vi "Mod_OFDM_Retrieve_Frame_Parameters.vi"(0 "Configuration in":variant, 11 "error in (no error)":errorcluster) -> (2 "Pulse Shaping Parameters":T2={"System Filter"={"TX Filter"=enum."Root Raised Cos", "Alpha"=0.5, "filter length"=8}, "Modulation system parameters"={"samples per symbol (16)"=16}, "symbol rate (Hz)"=1.0} {"symbol rate (Hz)" min=1.0 step=1.0 format="%.2p"; "Modulation system parameters"."samples per symbol (16)" step=2; "System Filter"."Alpha" min=0.0 max=1.0 step=0.05 format="%.2f"}, 4 "Parameters per Ofdm Symbol":T1 {"Data Source"."Data Source"."Register Initial State" format="%08x"}, 8 "Initial SEED IN":u32[](array[numeric]), 15 "error out":errorcluster)   [LabVIEW 2010]
doc: "The VI recovers the configuration settings from the variant into an array of clusters. The size of the array is the number of OFDM Symbols in the frame. Each cluster contains the configuration settings perataining to an OFDM symbol."
uses:
  Controls(Type_DEf)/Configure Pulse Shaping.ctl
  Controls(Type_DEf)/Parameters per Ofdm Symbol.ctl
  Polymorphic_Sub_VI's/Mod_OFDM_Get_OFDM_Frame.vi
  Polymorphic_Sub_VI's/Mod_OFDM_Get_Pulse_Shaping.vi
  Polymorphic_Sub_VI's/Mod_OFDM_Get_Data_Sources.vi
  Polymorphic_Sub_VI's/Mod_OFDM_Get_Modulator_Sources.vi
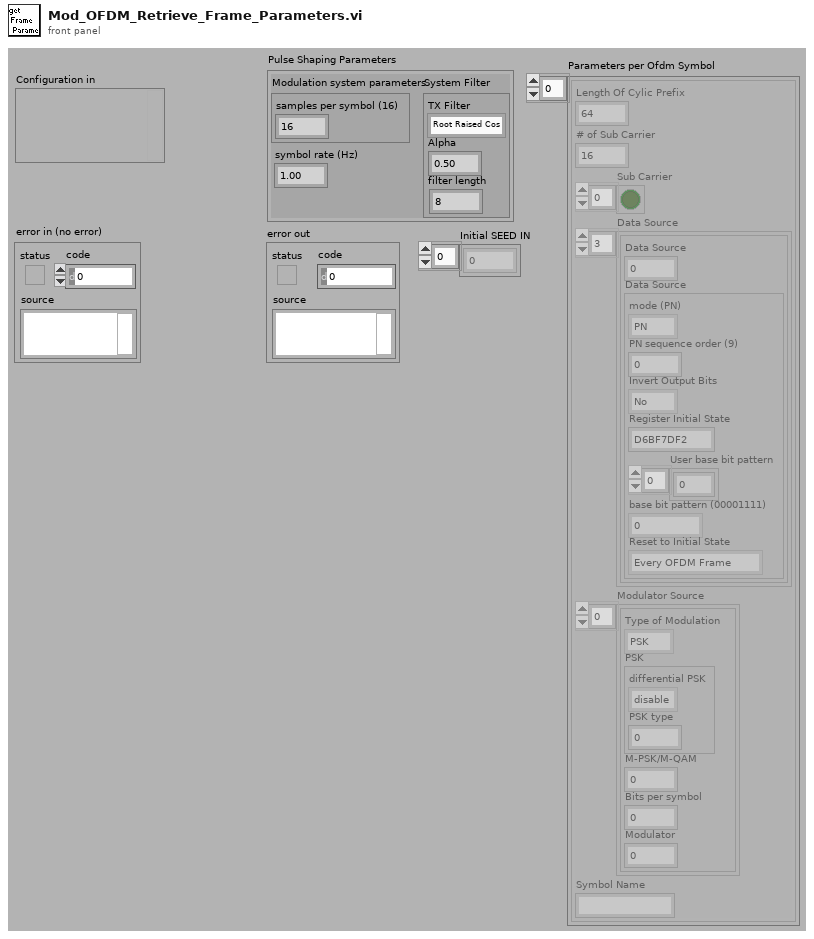
[diagram p1: front panel]
types:
  T1 = typedef "Parameters per Ofdm Symbol.ctl" = cluster{"Length Of Cylic Prefix":i32, "# of Sub Carrier":i32, "Sub Carrier":bool[], "Data Source":cluster{"Data Source":u16, "Data Source":cluster{"mode (PN)":enum16{"PN", "pattern", "user"}, "PN sequence order (9)":i32, "Invert Output Bits":enum16{"No", "Yes"}, "Register Initial State":u32, "User base bit pattern":i8[], "base bit pattern (00001111)":enum16{"0", "1", "01", "0011", "00001111"}, "Reset to Initial State":enum16{"Every OFDM Frame", "Every OFDM Symbol", "Every Sub Carrier"}}}[], "Modulator Source":cluster{"Type of Modulation":enum16{"PSK", "QAM"}, "PSK":cluster{"differential PSK":enum16{"disable", "enable"}, "PSK type":u16}, "M-PSK/M-QAM":i32, "Bits per symbol":i32, "Modulator":u16}[], "Symbol Name":string}[]
  T2 = typedef "Configure Pulse Shaping.ctl" = cluster{"System Filter":cluster{"TX Filter":enum16{"none", "Raised Cosine", "Root Raised Cos"}, "Alpha":dbl, "filter length":i32}, "Modulation system parameters":cluster{"samples per symbol (16)":u32}, "symbol rate (Hz)":dbl}
  T3 = cluster{"Symbol Name":string, "# of Symbols":i32}[]
  T4 = typedef "Pool of Data Source Control.ctl" = cluster{"mode (PN)":enum16{"PN", "pattern", "user"}, "PN sequence order (9)":i32, "Invert Output Bits":enum16{"No", "Yes"}, "Register Initial State ":u32, "User base bit pattern":i8[], "base bit pattern (00001111)":enum16{"0", "1", "01", "0011", "00001111"}, "Reset to Initial State":enum16{"Every OFDM Frame", "Every OFDM Symbol", "Every Sub Carrier"}}[]
  T5 = typedef "Pool of Modulator Control.ctl" = cluster{"M-QAM":enum16{"4", "16", "64", "256"}, "M-PSK":enum16{"2", "4", "8", "16", "32", "64", "128", "256"}, "Type of Modulation":enum16{"PSK", "QAM"}, " PSK":cluster{"differential PSK":enum16{"disable", "enable"}, "PSK type":enum16{"normal", "shifted", "offset"}}}[]
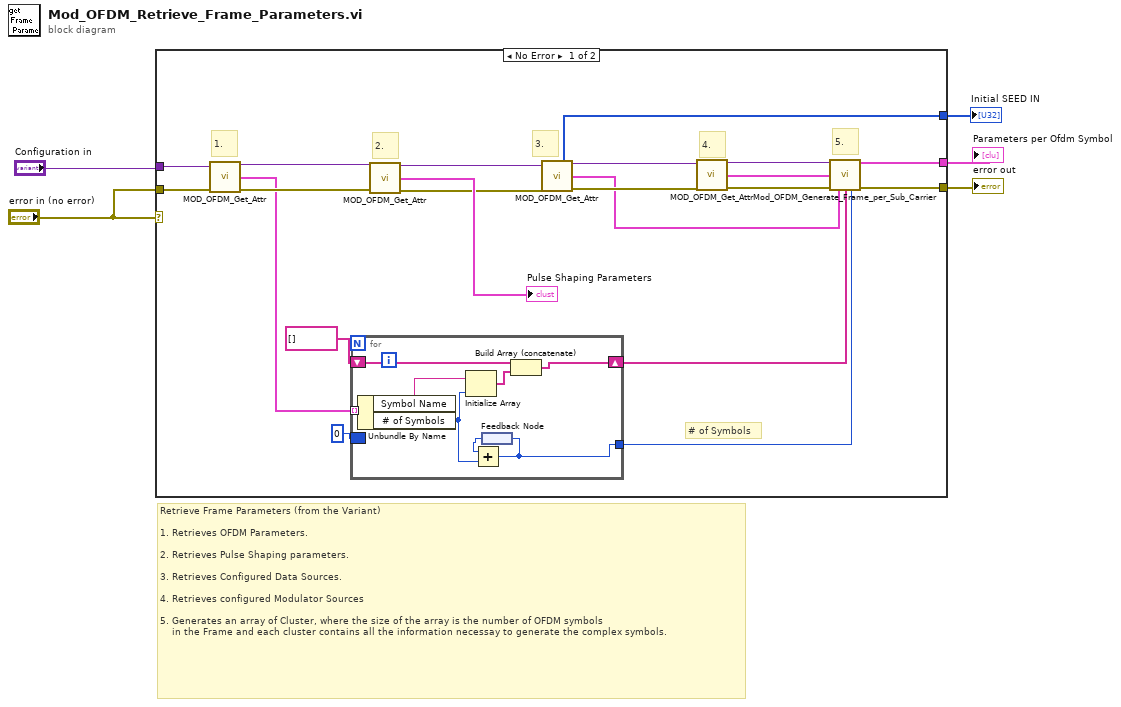
[diagram p0: block diagram]
diagram:
  # "Retrieve Frame Parameters (from the Variant)\n\n1. Retrieves OFDM Parameters.\n \n2. Retrieves Pulse Shaping parameters.\n\n3. Retrieves Configured Data Sources.\n\n4. Retrieves configured Modulator Sources\n\n5. Generates an array of Cluster, where the size of the array is the number of OFDM symbols\n    in the Frame and each cluster contains all the information necessay to generate the complex symbols."
  n1 = case shown="No Error" "error in (no error)" {
    tunnel: "Configuration in" -> [w26 _]
    tunnel: "error in (no error)" -> [w25 w35]
    tunnel: [w14 _] -> w4
    tunnel: [w13 w35] -> w3
    tunnel: [w9 _] -> w1
    frame No Error {
      # "# of Symbols"
      # "5."
      # "4."
      # "3."
      # "2."
      # "1."
      n2 = call-poly "MOD_OFDM_Get_Attr.vi"("Configuration in"=w26, "error in"=w25) -> ("Configuration out"=w23:variant, "OFDM Frame"=w17:T3, "error out"=w24:errorcluster)  [unwired: 10 in, 1 out]
      n3 = for {
        tunnel: w17 -> [w34] mode=indexing
        shift-right: [w32] -> w10
        shift-left: string[] [] -> [w30]
        tunnel: [w28] -> w7
        border: 0 -> [_]
        n4 = Unbundle By Name(w34) -> ("Symbol Name"=w33:string, "# of Symbols"=w27:i32)
        n5 = Initialize Array(w33, w27) -> (w31:string[])
        n6 = feedback #1() -> (w29:i32)
        n7 = Add(x=w29, y=w27) -> (x+y=w28:i32)
        n8 = feedback-in #1(w28) -> ()
        n9 = Build Array (concatenate)(w30, w31) -> (w32:string[])
      }
      n10 = call-poly "MOD_OFDM_Get_Attr.vi"("Configuration in"=w23, "error in"=w24) -> ("Configuration out"=w19:variant, "Pulse Shaping"=→"Pulse Shaping Parameters":T2, "error out"=w21:errorcluster)  [unwired: 10 in, 1 out]
      n11 = call-poly "MOD_OFDM_Get_Attr.vi"("Configuration in"=w19, "error in"=w21) -> ("Initial SEED IN"=w9:u32[], "Configuration out"=w18:variant, "Pool of Data Sources"=w11:T4, "error out"=w20:errorcluster)  [unwired: 7 in, 3 out]
      n12 = call-poly "MOD_OFDM_Get_Attr.vi"("Configuration in"=w18, "error in"=w20) -> ("Configuration out"=w15:variant, "Pool of Modulators"=w12:T5, "error out"=w16:errorcluster)  [unwired: 8 in, 3 out]
      n13 = call "Mod_OFDM_Generate_Frame_per_Sub_Carrier.vi"("Configure Variant"=w15, "Pool of Modulators"=w12, "error in"=w16, "Pool of Data Sources"=w11, "Symbol names in Frame"=w10, "# of Symbols"=w7) -> ("Parameters per OFDM Symbol"=w14:T1, "error out"=w13:errorcluster)  [unwired: 8 in]
    }
    frame Error {
    }
  }
  "Parameters per Ofdm Symbol" <- w4
  "error out" <- w3
  "Initial SEED IN" <- w1
